vi "Teleop.vi"(10 "Match Info":T1={"Autonomous Elapsed Seconds"=0.0, "TeleOp Elapsed Seconds"=0.0, "Disabled Elapsed Seconds"=0.0, "Visited Autonomous"=FALSE, "Visited TeleOp"=FALSE, "Visited Disabled"=FALSE, "Autonomous Settings"={"Autonomous Style"=enum."Independent", "VI Refnum"=refnum}}, 11 "Call Context":T2) -> ()   [LabVIEW 2014]
doc: "This VI is called for each TeleOp packet received from the DS where the robot is not disabled. It is often used to read from the joysticks and update I/O or to update setpoints for timed control loops. It should complete and return within 20 milliseconds or it may miss DS packets."
uses:
  <vilib>/Rock Robotics/WPI/DriverStation/WPI_DriverStationDerivedRobotMode.ctl
  <vilib>/Rock Robotics/WPI/DriverStation/WPI_DriverStationMatch Info.ctl
  <vilib>/Rock Robotics/WPI/Solenoid/WPI_SolenoidValue.ctl
  <vilib>/Rock Robotics/WPI/RobotDrive/WPI_RobotDriveGetSetRefNum.vi
  <vilib>/Rock Robotics/WPI/Joystick/WPI_JoystickGetSetRefNum.vi
  <vilib>/Rock Robotics/Network Tables/SD Write Boolean Array.vi
  <vilib>/Rock Robotics/Network Tables/SD Write Numeric Array.vi
  <vilib>/Rock Robotics/Network Tables/SD Read Boolean.vi
  <vilib>/Rock Robotics/Network Tables/SD Read Number.vi
  <vilib>/Rock Robotics/WPI/Solenoid/WPI_SolenoidSetEnum.vi
  Labview files/swerve drive library/Pivot Library Test/Pivot Drive.lvlib
panel:
  out "Sample Slider 0":dbl(slide) scale=0.0..5.0
  out "Sample Boolean 1":bool
  out "Sample Boolean 0":bool
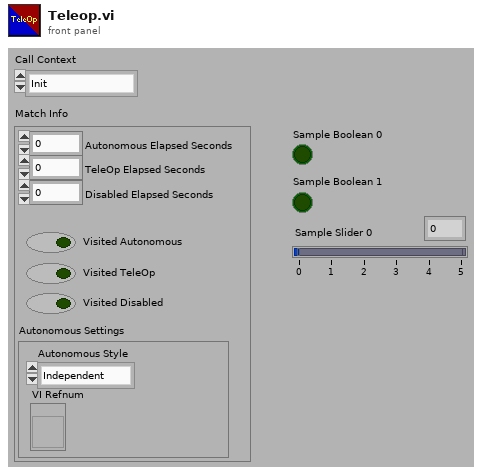
[diagram p1: front panel]
types:
  T1 = typedef "WPI_DriverStationMatch Info.ctl" = cluster{"Autonomous Elapsed Seconds":dbl, "TeleOp Elapsed Seconds":dbl, "Disabled Elapsed Seconds":dbl, "Visited Autonomous":bool, "Visited TeleOp":bool, "Visited Disabled":bool, "Autonomous Settings":cluster{"Autonomous Style":enum16{"Iterative", "Independent"}, "VI Refnum":refnum<vi>}}
  T2 = typedef "WPI_DriverStationDerivedRobotMode.ctl" = enum16{"Init", "Execute", "Stop"}
  T3 = typedef "WPI_SolenoidValue.ctl" = enum16{"Off", "On", "Forward", "Reverse"}
  T4 = typedef "WPI_EncoderDevRef.ctl" = cluster{"DevStatus":errorcluster, "EncoderIndex":T5, "CounterIndex":T6, "DistancePerCount":dbl, "Decoding Type":T7}
  T5 = typedef "FPGA_EncoderIdx.ctl" = enum8{"Enc 0", "Enc 1", "Enc 2", "Enc 3", "Enc 4", "Enc 5", "Enc 6", "Enc 7", "Invalid"}
  T6 = typedef "FPGA_CounterCtrSystemIndex.ctl" = enum8{"Ctr 0", "Ctr 1", "Ctr 2", "Ctr 3", "Ctr 4", "Ctr 5", "Ctr 6", "Ctr 7", "Invalid"}
  T7 = typedef "WPI_EncoderType.ctl" = enum16{"1x", "2x", "4x"}
  T8 = typedef "WPI_RobotDriveDevRef.ctl" = cluster{"DevStatus":errorcluster, "Motors[]":T9[], "Square Inputs":bool, "Max Output":dbl}
  T9 = typedef "WPI_MotorControlDeviceRef.ctl" = cluster{"DeviceStatus":errorcluster, "Type":T10, "PWM":cluster{"Controller":T11, "PWM Channel":T12, "DeadBand":T13}, "CAN":cluster{"Device Number":u8, "Control Mode":T14, "Semaphore":T15, "Max Vout":dbl, "TalonSRX Control Mode":T16}, "Invert":bool, "TransformRef":T17, "InvTransformRef":T17}
  T10 = typedef "WPI_MotorControlType.ctl" = enum16{"PWM", "CAN", "CANTalonSRX"}
  T11 = typedef "FPGA_TypedefDigitalModule.ctl" = enum16{"Controller 1"}
  T12 = typedef "FPGA_DIOPWMChannel.ctl" = enum8{"PWM 0", "PWM 1", "PWM 2", "PWM 3", "PWM 4", "PWM 5", "PWM 6", "PWM 7", "PWM 8", "PWM 9", "PWM MXP 0", "PWM MXP 1", "PWM MXP 2", "PWM MXP 3", "PWM MXP 4", "PWM MXP 5", "PWM MXP 6", "PWM MXP 7", "PWM MXP 8", "PWM MXP 9", "Invalid"}
  T13 = typedef "WPI_PWMDeadband.ctl" = cluster{"Name":string, "maxPositivePwm":i32, "minPositivePwm":i32, "centerPwm":i32, "maxNegativePwm":i32, "minNegativePwm":i32, "angularRange":u16}
  T14 = typedef "WPI_CANJaguar_ControlMode.ctl" = enum8{"Percent VBus", "Current", "Speed", "Position", "Voltage"}
  T15 = typedef "Semaphore RefNum" = refnum<k1>
  T16 = typedef "WPI_CANTalonSRX_APIControlMode.ctl" = enum8{"Percent VBus", "Speed", "Position", "Slave", "Unchanged / Invalid"}
  T17 = typedef "WPI_PWMTransform_ConPane.ctl" = refnum<vi>
  T18 = typedef "WPI_JoystickDevRef.ctl" = cluster{"Device":T19}
  T19 = typedef "WPI_JoystickDeviceEnum.ctl" = enum16{"USB 0", "USB 1", "USB 2", "USB 3", "USB 4", "USB 5"}
  T20 = typedef "WPI_DigitalInputDevRef.ctl" = cluster{"DevStatus":errorcluster, "DIO Channel":T21, "Controller":T11}
  T21 = typedef "FPGA_DIOChannel.ctl" = enum8{"DIO 0", "DIO 1", "DIO 2", "DIO 3", "DIO 4", "DIO 5", "DIO 6", "DIO 7", "DIO 8", "DIO 9", "DIO MXP 0", "DIO MXP 1", "DIO MXP 2", "DIO MXP 3", "DIO MXP 4", "DIO MXP 5", "DIO MXP 6", "DIO MXP 7", "DIO MXP 8", "DIO MXP 9", "DIO MXP 10", "DIO MXP 11", "DIO MXP 12", "DIO MXP 13", "DIO MXP 14", "DIO MXP 15", "Invalid"}
  T22 = typedef "WPI_SolenoidDevRef.ctl" = cluster{"DevStatus":errorcluster, "Pneumatics Control Module":u8, "Forward Solenoid Channel":T23, "Reverse Solenoid Channel":T23}
  T23 = typedef "WPI_SolenoidChannel.ctl" = enum8{"Solenoid 0", "Solenoid 1", "Solenoid 2", "Solenoid 3", "Solenoid 4", "Solenoid 5", "Solenoid 6", "Solenoid 7", "Invalid"}
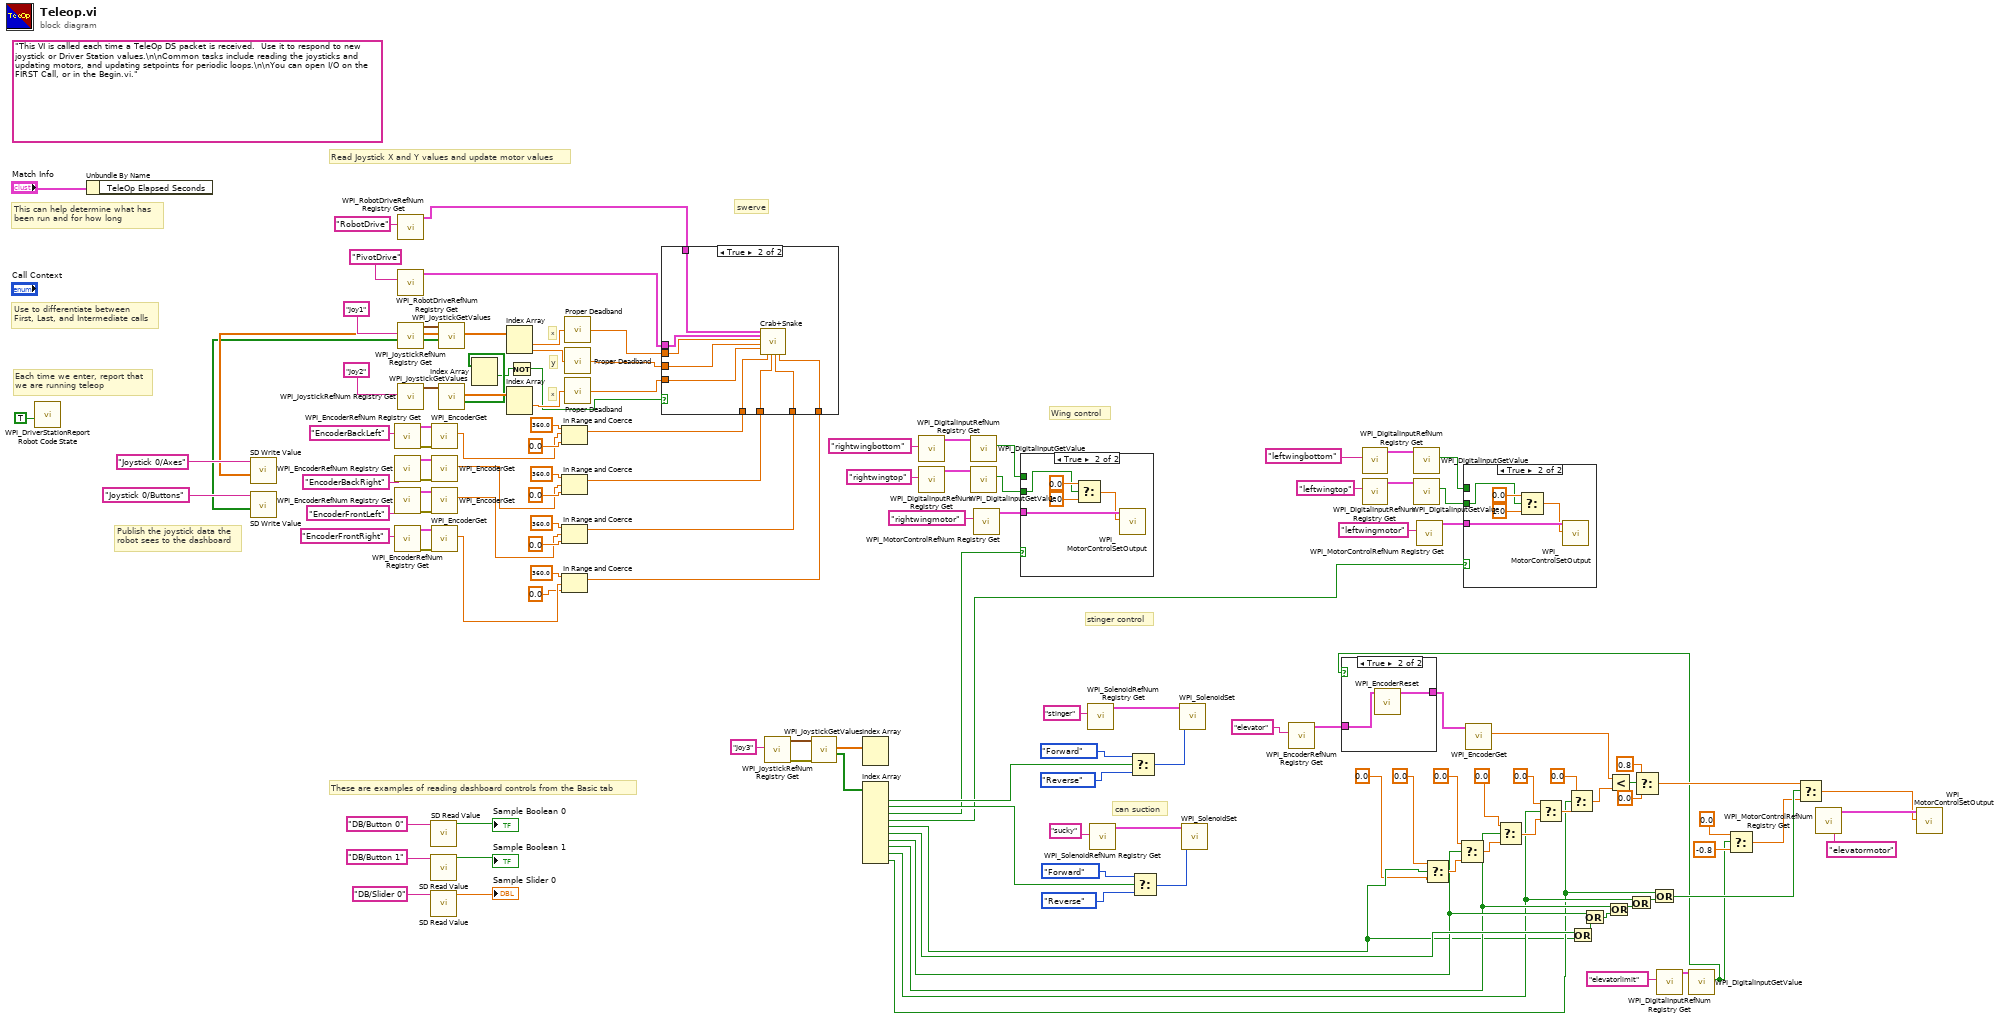
[diagram p0: block diagram]
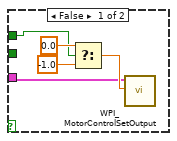
[diagram p3: hidden frame]
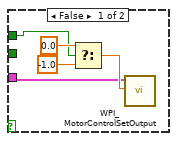
[diagram p4: hidden frame]
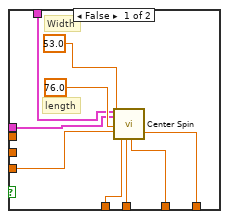
[diagram p5: hidden frame]
diagram:
  (unwired) "This VI is called each time a TeleOp DS packet is received.  Use it to respond to new joystick or Driver Station values.\n\nCommon tasks include reading the joysticks and updating motors, and updating setpoints for periodic loops.\n\nYou can open I/O on the FIRST Call, or in the Begin.vi."
  # "swerve"
  # "Wing control"
  # "stinger control"
  # "can suction"
  # "x"
  # "y"
  # "x"
  # "These are examples of reading dashboard controls from the Basic tab"
  # "Publish the joystick data the\nrobot sees to the dashboard"
  # "Each time we enter, report that\nwe are running teleop"
  # "Use to differentiate between\nFirst, Last, and Intermediate calls"
  # "This can help determine what has\nbeen run and for how long"
  # "Read Joystick X and Y values and update motor values"
  n1 = call <vilib>:"WPI_DriverStationReport Robot Code State.vi"("TeleOp"=TRUE ("Autonomous")) -> ()  [unwired: 10 in, 1 out]
  n2 = Unbundle By Name("Match Info") -> ()  [unwired: 1 out]
  n3 = call <vilib>:"WPI_EncoderRefNum Registry Get.vi"("refnum name"="EncoderBackLeft") -> ("error out"=w107:errorcluster, "EncoderDevRef"=w106:T4)  [unwired: 9 in]
  n4 = call <vilib>:"WPI_EncoderRefNum Registry Get.vi"("refnum name"="EncoderBackRight") -> ("error out"=w105:errorcluster, "EncoderDevRef"=w104:T4)  [unwired: 9 in]
  n5 = call <vilib>:"WPI_EncoderRefNum Registry Get.vi"("refnum name"="EncoderFrontLeft") -> ("error out"=w103:errorcluster, "EncoderDevRef"=w102:T4)  [unwired: 9 in]
  n6 = call <vilib>:"WPI_EncoderRefNum Registry Get.vi"("refnum name"="EncoderFrontRight") -> ("error out"=w101:errorcluster, "EncoderDevRef"=w100:T4)  [unwired: 9 in]
  n7 = call <vilib>:"WPI_RobotDriveRefNum Registry Get.vi"("refnum name"="PivotDrive") -> ("RobotDriveDevRef"=w78:T8)  [unwired: 1 in, 9 out]
  n8 = call <vilib>:"WPI_JoystickRefNum Registry Get.vi"("refnum name"="Joy1") -> ("JoystickDevRef"=w129:T18)  [unwired: 1 in, 9 out]
  n9 = call <vilib>:"WPI_JoystickRefNum Registry Get.vi"("refnum name"="Joy2") -> ("JoystickDevRef"=w113:T18)  [unwired: 1 in, 9 out]
  n10 = call <vilib>:"WPI_RobotDriveRefNum Registry Get.vi"("refnum name"="RobotDrive") -> ("RobotDriveDevRef"=w79:T8)  [unwired: 9 in, 1 out]
  n11 = call-poly <vilib>:"SD Read Value.vi"("Name"="DB/Button 0" ("refnum name")) -> ("Boolean"=→"Sample Boolean 0":bool)  [unwired: 8 in, 2 out]
  n12 = call-poly <vilib>:"SD Read Value.vi"("Name"="DB/Button 1" ("refnum name")) -> ("Boolean"=→"Sample Boolean 1":bool)  [unwired: 8 in, 2 out]
  n13 = call-poly <vilib>:"SD Read Value.vi"("Name"="DB/Slider 0" ("refnum name")) -> ("Numeric"=→"Sample Slider 0":dbl)  [unwired: 8 in, 2 out]
  n14 = call <vilib>:"WPI_EncoderGet.vi"("error in (no error)"=w107, "EncoderDevRef"=w106) -> ("Distance"=w92:dbl)  [unwired: 9 out]
  n15 = call <vilib>:"WPI_EncoderGet.vi"("error in (no error)"=w105, "EncoderDevRef"=w104) -> ("Distance"=w91:dbl)  [unwired: 9 out]
  n16 = call <vilib>:"WPI_EncoderGet.vi"("error in (no error)"=w103, "EncoderDevRef"=w102) -> ("Distance"=w90:dbl)  [unwired: 9 out]
  n17 = call <vilib>:"WPI_EncoderGet.vi"("error in (no error)"=w101, "EncoderDevRef"=w100) -> ("Distance"=w89:dbl)  [unwired: 9 out]
  n18 = call <vilib>:"WPI_JoystickGetValues.vi"("JoystickDevRef"=w129) -> ("Buttons"=w118:bool[], "Axes"=w120:dbl[])  [unwired: 6 in, 3 out]
  n19 = call-poly <vilib>:"SD Write Value.vi"("Numeric Array"=w120, "Name"="Joystick 0/Axes") -> ()  [unwired: 8 in, 2 out]
  n20 = call-poly <vilib>:"SD Write Value.vi"("Boolean Array"=w118, "Name"="Joystick 0/Buttons") -> ()  [unwired: 8 in, 2 out]
  n21 = call <vilib>:"WPI_JoystickGetValues.vi"("JoystickDevRef"=w113) -> ("Buttons"=w88:bool[], "Axes"=w114:dbl[])  [unwired: 6 in, 3 out]
  n22 = Index Array(array=w88) -> (element #1=w87:bool)  [unwired: 2 in, 1 out]
  n23 = Index Array(array=w120) -> (element #1=w116:dbl, element #2=w117:dbl)  [unwired: 2 in]
  n24 = Index Array(array=w114) -> (element #1=w115:dbl)  [unwired: 2 in, 1 out]
  n25 = Not(x=w87) -> (.not. x?=w86:bool)
  n26 = In Range and Coerce(upper limit=360.0, x=w92, lower limit=0.0 ("upper limit")) -> (coerced(x)=w82:dbl)  [unwired: 1 out]
  n27 = In Range and Coerce(upper limit=360.0, x=w91, lower limit=0.0 ("upper limit")) -> (coerced(x)=w83:dbl)  [unwired: 1 out]
  n28 = In Range and Coerce(upper limit=360.0, x=w90, lower limit=0.0 ("upper limit")) -> (coerced(x)=w84:dbl)  [unwired: 1 out]
  n29 = In Range and Coerce(upper limit=360.0, x=w89, lower limit=0.0 ("upper limit")) -> (coerced(x)=w85:dbl)  [unwired: 1 out]
  n30 = call "Proper Deadband.vi"("Value"=w116) -> ("Deadbanded Value"=w77:dbl)
  n31 = call "Proper Deadband.vi"("Value"=w117) -> ("Deadbanded Value"=w76:dbl)
  n32 = call "Proper Deadband.vi"("Value"=w115) -> ("Deadbanded Value"=w81:dbl)
  n33 = case shown="True" w86 {
    tunnel: w85 -> [w141 w150]
    tunnel: w84 -> [w140 w149]
    tunnel: w83 -> [w139 w148]
    tunnel: w82 -> [w138 w147]
    tunnel: w81 -> [w137 w143]
    tunnel: w79 -> [w134 w146]
    tunnel: w78 -> [w133 w145]
    tunnel: w77 -> [_ w144]
    tunnel: w76 -> [_ w142]
    frame False {
      # "Width"
      # "length"
      n34 = call "Center Spin.vi"("RobotDriveDevRef"=w134, "RobotPivotDevRef"=w133, "Width"=53.0, "Legnth"=76.0, "Joystick axis"=w137, "Rear Left Current Pivot Angle"=w138, "Rear Right Current Pivot Angle"=w139, "Front Left Current Pivot Angle"=w140, "Front Right Current Pivot Angle"=w141) -> ()  [unwired: 8 in, 3 out]
    }
    frame True {
      n35 = call "Crab+Snake.vi"("RobotDriveDevRef"=w146, "RobotPivotDevRef"=w145, "Joystick 1 X"=w144, "Joystick 1 Y"=w142, "Joystick 2 X"=w143, "Rear Left Current Pivot Angle"=w147, "Rear Right Current Pivot Angle"=w148, "Front Left Current Pivot Angle"=w149, "Front Right Current Pivot Angle"=w150) -> ()  [unwired: 1 in, 10 out]
    }
  }
  n36 = call <vilib>:"WPI_JoystickRefNum Registry Get.vi"("refnum name"="Joy3") -> ("error out"=w74:errorcluster, "JoystickDevRef"=w73:T18)  [unwired: 9 in]
  n37 = call <vilib>:"WPI_JoystickGetValues.vi"("error in (no error)"=w74, "JoystickDevRef"=w73) -> ("Buttons"=w71:bool[], "Axes"=w72:dbl[])  [unwired: 5 in, 3 out]
  n38 = Index Array(array=w72) -> ()  [unwired: 2 in, 2 out]
  n39 = Index Array(array=w71) -> (element #1=w68:bool, element #2=w59:bool, element #3=w57:bool, element #4=w40:bool, element #5=w2:bool, element #6=w13:bool, element #7=w12:bool, element #8=w11:bool, element #9=w10:bool, element #10=w9:bool)  [unwired: 10 in]
  n40 = call <vilib>:"WPI_DigitalInputRefNum Registry Get.vi"("refnum name"="rightwingbottom") -> ("DigitalInputDevRef"=w53:T20)  [unwired: 9 in, 1 out]
  n41 = call <vilib>:"WPI_DigitalInputRefNum Registry Get.vi"("refnum name"="rightwingtop") -> ("DigitalInputDevRef"=w52:T20)  [unwired: 9 in, 1 out]
  n42 = call <vilib>:"WPI_DigitalInputGetValue.vi"("DigitalInputDevRef"=w53) -> ("Value"=w54:bool)  [unwired: 8 in, 2 out]
  n43 = call <vilib>:"WPI_DigitalInputGetValue.vi"("DigitalInputDevRef"=w52) -> ("Value"=w55:bool)  [unwired: 8 in, 2 out]
  n44 = call <vilib>:"WPI_MotorControlRefNum Registry Get.vi"("refnum name"="rightwingmotor") -> ("MotorControlDevRef"=w56:T9)  [unwired: 9 in, 1 out]
  n45 = case shown="True" w57 {
    tunnel: w56 -> [w152 w160]
    tunnel: w55 -> [_ w156]
    tunnel: w54 -> [w151 _]
    frame False {
      n46 = Select(t=0.0, s=w151, f=-1.0) -> (s? t:f=w155:dbl)
      n47 = call <vilib>:"WPI_MotorControlSetOutput.vi"("Output"=w155, "MotorControlDevRef"=w152) -> ()  [unwired: 7 in, 3 out]
    }
    frame True {
      n48 = Select(t=0.0, s=w156, f=1.0) -> (s? t:f=w159:dbl)
      n49 = call <vilib>:"WPI_MotorControlSetOutput.vi"("Output"=w159, "MotorControlDevRef"=w160) -> ()  [unwired: 7 in, 3 out]
    }
  }
  n50 = call <vilib>:"WPI_SolenoidRefNum Registry Get.vi"("refnum name"="stinger") -> ("SolenoidDevRef"=w66:T22)  [unwired: 9 in, 1 out]
  n51 = call <vilib>:"WPI_SolenoidRefNum Registry Get.vi"("refnum name"="sucky") -> ("SolenoidDevRef"=w63:T22)  [unwired: 9 in, 1 out]
  n52 = Select(t=WPI_SolenoidValue."Forward" ("Value"), s=w68, f=WPI_SolenoidValue."Reverse" ("Value")) -> (s? t:f=w67:T3)
  n53 = Select(t=WPI_SolenoidValue."Forward" ("Value"), s=w59, f=WPI_SolenoidValue."Reverse" ("Value")) -> (s? t:f=w62:T3)
  n54 = call-poly <vilib>:"WPI_SolenoidSet.vi"("Value"=w67, "SolenoidDevRef"=w66) -> ()  [unwired: 1 in, 9 out]
  n55 = call-poly <vilib>:"WPI_SolenoidSet.vi"("Value"=w62, "SolenoidDevRef"=w63) -> ()  [unwired: 1 in, 9 out]
  n56 = call <vilib>:"WPI_EncoderRefNum Registry Get.vi"("refnum name"="elevator") -> ("EncoderDevRef"=w8:T4)  [unwired: 9 in, 1 out]
  n57 = call <vilib>:"WPI_DigitalInputRefNum Registry Get.vi"("refnum name"="leftwingbottom") -> ("DigitalInputDevRef"=w44:T20)  [unwired: 9 in, 1 out]
  n58 = call <vilib>:"WPI_DigitalInputRefNum Registry Get.vi"("refnum name"="leftwingtop") -> ("DigitalInputDevRef"=w45:T20)  [unwired: 9 in, 1 out]
  n59 = call <vilib>:"WPI_DigitalInputGetValue.vi"("DigitalInputDevRef"=w44) -> ("Value"=w43:bool)  [unwired: 8 in, 2 out]
  n60 = call <vilib>:"WPI_DigitalInputGetValue.vi"("DigitalInputDevRef"=w45) -> ("Value"=w42:bool)  [unwired: 8 in, 2 out]
  n61 = call <vilib>:"WPI_MotorControlRefNum Registry Get.vi"("refnum name"="leftwingmotor") -> ("MotorControlDevRef"=w41:T9)  [unwired: 9 in, 1 out]
  n62 = Select(t=0.0, s=w2, f=0.0 ("t")) -> (s? t:f=w32:dbl)
  n63 = Select(t=0.0, s=w12, f=w32) -> (s? t:f=w33:dbl)
  n64 = case shown="True" w40 {
    tunnel: w41 -> [w162 w170]
    tunnel: w42 -> [_ w166]
    tunnel: w43 -> [w161 _]
    frame False {
      n65 = Select(t=0.0, s=w161, f=-1.0) -> (s? t:f=w165:dbl)
      n66 = call <vilib>:"WPI_MotorControlSetOutput.vi"("Output"=w165, "MotorControlDevRef"=w162) -> ()  [unwired: 7 in, 3 out]
    }
    frame True {
      n67 = Select(t=0.0, s=w166, f=1.0) -> (s? t:f=w169:dbl)
      n68 = call <vilib>:"WPI_MotorControlSetOutput.vi"("Output"=w169, "MotorControlDevRef"=w170) -> ()  [unwired: 7 in, 3 out]
    }
  }
  n69 = Select(t=0.0, s=w11, f=w33) -> (s? t:f=w34:dbl)
  n70 = Select(t=0.0, s=w10, f=w34) -> (s? t:f=w31:dbl)
  n71 = Select(t=0.0, s=w9, f=w31) -> (s? t:f=w30:dbl)
  n72 = Or(x=w13, y=w2) -> (x .or. y?=w14:bool)
  n73 = Or(x=w12, y=w14) -> (x .or. y?=w16:bool)
  n74 = Or(x=w11, y=w16) -> (x .or. y?=w15:bool)
  n75 = Or(x=w10, y=w15) -> (x .or. y?=w17:bool)
  n76 = Or(x=w9, y=w17) -> (x .or. y?=w22:bool)
  n77 = call <vilib>:"WPI_DigitalInputRefNum Registry Get.vi"("refnum name"="elevatorlimit") -> ("DigitalInputDevRef"=w24:T20)  [unwired: 9 in, 1 out]
  n78 = call <vilib>:"WPI_DigitalInputGetValue.vi"("DigitalInputDevRef"=w24) -> ("Value"=w6:bool)  [unwired: 8 in, 2 out]
  n79 = case shown="True" w6 {
    tunnel: [w171 w173] -> w7
    tunnel: w8 -> [w171 w172]
    frame False {
    }
    frame True {
      n80 = call <vilib>:"WPI_EncoderReset.vi"("EncoderDevRef"=w172) -> ("EncoderDevRef"=w173:T4)  [unwired: 1 in, 9 out]
    }
  }
  n81 = call <vilib>:"WPI_EncoderGet.vi"("EncoderDevRef"=w7) -> ("Distance"=w37:dbl)  [unwired: 1 in, 9 out]
  n82 = Less?(x=w37, y=w30) -> (x < y?=w38:bool)
  n83 = Select(t=0.8, s=w38, f=0.0) -> (s? t:f=w18:dbl)
  n84 = Select(t=0.0, s=w6, f=-0.8) -> (s? t:f=w19:dbl)
  n85 = Select(t=w18, s=w22, f=w19) -> (s? t:f=w4:dbl)
  n86 = call <vilib>:"WPI_MotorControlRefNum Registry Get.vi"("refnum name"="elevatormotor") -> ("MotorControlDevRef"=w5:T9)  [unwired: 9 in, 1 out]
  n87 = call <vilib>:"WPI_MotorControlSetOutput.vi"("Output"=w4, "MotorControlDevRef"=w5) -> ()  [unwired: 7 in, 3 out]
